vi "qerryPos.vi"(3 "error in (no error)":errorcluster, 6 "UART in":refnum<visa-resource-name>) -> (0 "error out":errorcluster, 1 "Array":dbl[](array[numeric]), 2 "UART out":refnum<visa-resource-name>)   [LabVIEW 2016]
panel:
  out "Numeric":dbl
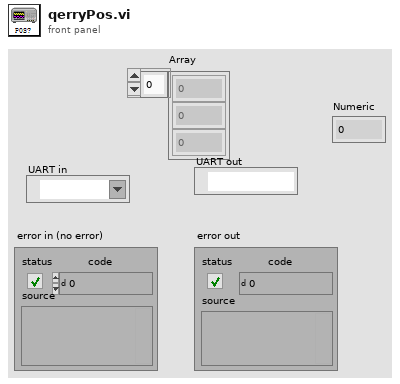
[diagram p1: front panel]
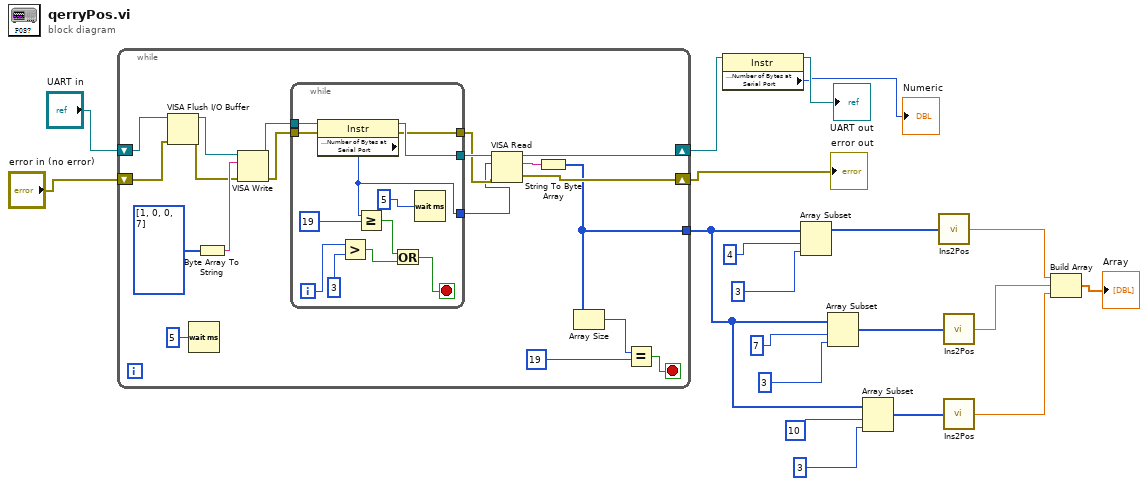
[diagram p0: block diagram]
diagram:
  n1 = while {
    shift-right: [w33] -> w3
    shift-left: "UART in" -> [w26]
    shift-right: [w32] -> w4
    shift-left: "error in (no error)" -> [w25]
    tunnel: [w31] -> w11
    stop <- w36 stop-if-true
    n2 = VISA Flush I/O Buffer(VISA resource name=w26, error in (no error)=w25) -> (VISA resource name out=w24:refnum<visa-resource-name>, error out=w23:errorcluster)  [unwired: 1 in]
    n3 = Wait (ms)(milliseconds to wait=u32 5) -> ()  [unwired: 1 out]
    n4 = Byte Array To String(unsigned byte array=i32[] [1, 0, 0, 7]) -> (string=w38:string)
    n5 = VISA Write(VISA resource name=w24, write buffer=w38, error in (no error)=w23) -> (VISA resource name out=w29:refnum<visa-resource-name>, error out=w30:errorcluster)  [unwired: 1 out]
    n6 = while {
      tunnel: w30 -> [w51]
      tunnel: w29 -> [w50]
      tunnel: [w48] -> w28
      tunnel: [w47] -> w27
      tunnel: [w40] -> w22
      i -> [w45]
      stop <- w41 stop-if-true
      n7 = property class="Instr"(reference=w50, error in=w51) -> (reference out=w48:refnum<visa-resource-name>, error out=w47:errorcluster, "Serial Settings:Number of Bytes at Serial Port"=w40:u32)
      n8 = Greater?(x=w45, y=3) -> (0:w42:bool)
      n9 = Greater Or Equal?(x=w40, y=19) -> (x >= y?=w43:bool)
      n10 = Or(x=w43, y=w42) -> (x .or. y?=w41:bool)
      n11 = Wait (ms)(milliseconds to wait=5) -> ()  [unwired: 1 out]
    }
    n12 = VISA Read(VISA resource name=w28, byte count=w22, error in (no error)=w27) -> (VISA resource name out=w33:refnum<visa-resource-name>, read buffer=w37:string, error out=w32:errorcluster)  [unwired: 1 out]
    n13 = String To Byte Array(string=w37) -> (unsigned byte array=w31:u8[])
    n14 = Array Size(array=w31) -> (size(s)=w35:i32)
    n15 = Equal?(x=w35, y=19) -> (x = y?=w36:bool)
  }
  "error out" <- w4
  n16 = property class="Instr"(reference=w3) -> (reference out=→"UART out":refnum<visa-resource-name>, "Serial Settings:Number of Bytes at Serial Port"=→"Numeric":u32)  [unwired: 1 in, 1 out]
  n17 = Array Subset(array=w11, index=4, length=3) -> (w16:u8[])
  n18 = Array Subset(array=w11, index=7, length=3) -> (w9:u8[])
  n19 = Array Subset(array=w11, index=10, length=3) -> (w10:u8[])
  n20 = call "Ins2Pos.vi"("Ins"=w16) -> ("Pos"=w8:dbl)
  n21 = call "Ins2Pos.vi"("Ins"=w9) -> ("Pos"=w7:dbl)
  n22 = call "Ins2Pos.vi"("Ins"=w10) -> ("Pos"=w6:dbl)
  n23 = Build Array(w8, w7, w6) -> (→"Array":dbl[])
